vi "teste._01vi.vi"() -> ()   [LabVIEW 2016]
panel:
  out "Array 2":dbl[](array[numeric])
  out "Array":dbl[](array[numeric])
  in  "Histórico":dbl[][][](array[numeric])
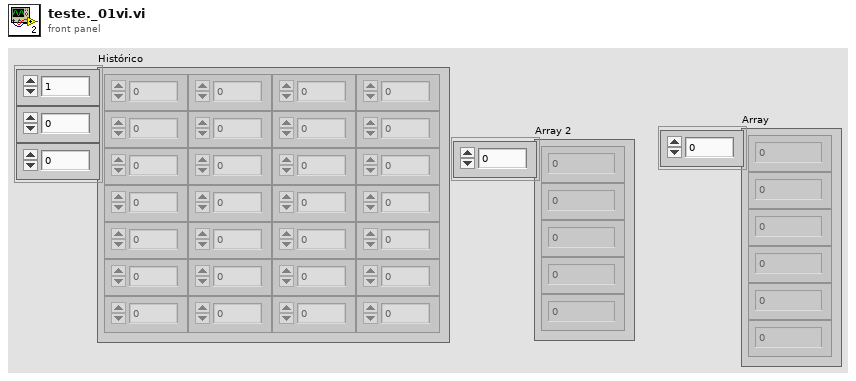
[diagram p1: front panel]
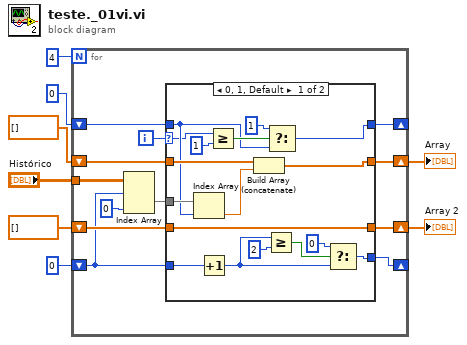
[diagram p0: block diagram]
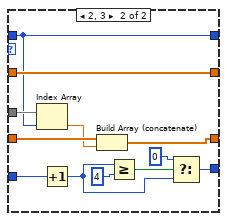
[diagram p2: hidden frame]
diagram:
  n1 = for {
    N: 4 -> [_]
    tunnel: "Histórico" -> [w13]
    shift-right: [w19] -> _
    shift-left: 0 -> [w20]
    shift-right: [w16] -> w5
    shift-left: dbl[] [] -> [w17]
    shift-right: [w14] -> w4
    shift-left: dbl[] [] -> [w15]
    shift-right: [w10] -> _
    shift-left: 0 -> [w11]
    i -> [w18]
    n2 = Index Array(array=w13, index (dim 0)=w11, index (dim 2)=0 ("disabled index (col)")) -> (element=w12:dbl[])  [unwired: 1 in]
    n3 = case shown="0, 1, Default" w18 {
      selector: w18 -> [w21 _]
      tunnel: w12 -> [w37 w49]
      tunnel: w20 -> [w23 w38]
      tunnel: [w22 w38] -> w19
      tunnel: w17 -> [w35 w48]
      tunnel: [w36 w48] -> w16
      tunnel: w15 -> [w33 w47]
      tunnel: [w33 w45] -> w14
      tunnel: w11 -> [w32 w42]
      tunnel: [w27 w39] -> w10
      frame 0, 1, Default {
        n4 = Index Array(array=w37, index=w23) -> (element=w34:dbl)
        n5 = Increment(x=w32) -> (x+1=w28:i32)
        n6 = Greater Or Equal?(x=w21, y=1) -> (x >= y?=w25:bool)
        n7 = Build Array (concatenate)(w35, w34) -> (w36:dbl[])
        n8 = Greater Or Equal?(x=w28, y=2) -> (x >= y?=w30:bool)
        n9 = Select(t=1 ("y"), s=w25, f=w23) -> (s? t:f=w22:i32)
        n10 = Select(t=0 ("y"), s=w30, f=w28) -> (s? t:f=w27:i32)
      }
      frame 2, 3 {
        n11 = Index Array(array=w49, index=w38) -> (element=w46:dbl)
        n12 = Increment(x=w42) -> (x+1=w40:i32)
        n13 = Build Array (concatenate)(w47, w46) -> (w45:dbl[])
        n14 = Greater Or Equal?(x=w40, y=4) -> (x >= y?=w43:bool)
        n15 = Select(t=0 ("y"), s=w43, f=w40) -> (s? t:f=w39:i32)
      }
    }
  }
  "Array" <- w5
  "Array 2" <- w4
